vi "getNormLUT.vi"() -> ()   [LabVIEW 2012]
panel:
  in  "Number of Entries in LUT":dbl=512.0
  out "Init Data Out":u32[](array[numeric])
  in  "Frequency":dbl=1000.0
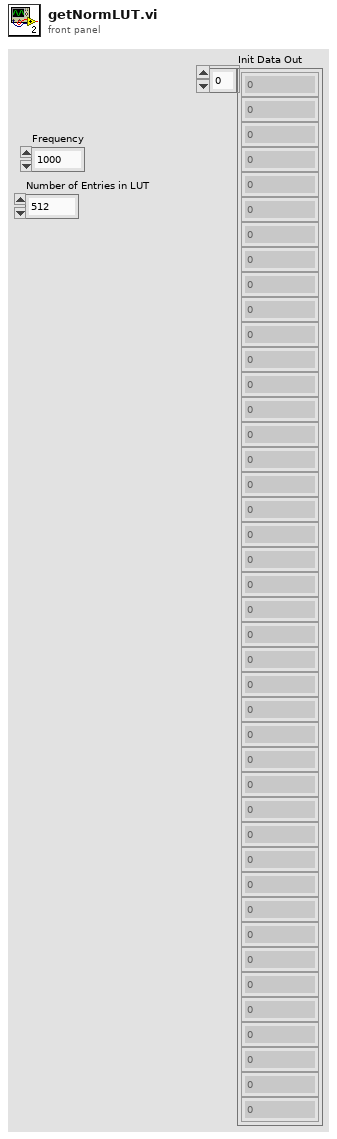
[diagram p1: front panel]
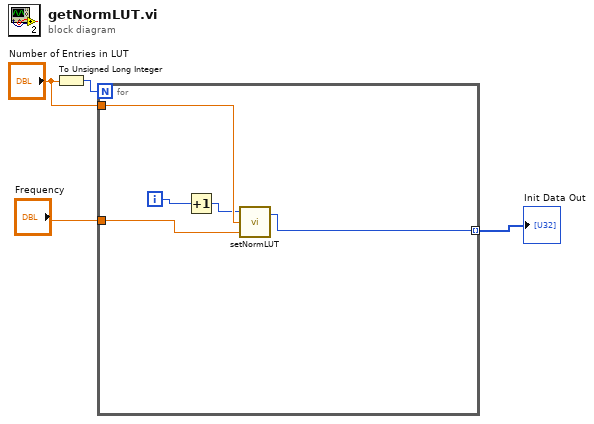
[diagram p0: block diagram]
diagram:
  n1 = To Unsigned Long Integer(number="Number of Entries in LUT") -> (unsigned 32bit integer=w1:u32)
  n2 = for {
    N: w1 -> [_]
    tunnel: "Frequency" -> [w9]
    tunnel: [w5] -> w3 mode=indexing
    tunnel: "Number of Entries in LUT" -> [w8]
    i -> [w7]
    n3 = Increment(x=w7) -> (x+1=w6:i32)
    n4 = call "setNormLUT.vi"("Frequency"=w9, "Number of entries in LUT"=w8, "Count"=w6) -> ("Normalized bin"=w5:u32)  [unwired: 1 out]
  }
  "Init Data Out" <- w3
